vi "processCmd.vi"(8 "error in (no error)":errorcluster, 10 "tcpPacket":T1, 11 "tcpServerCmd in":refnum<class "TcpServerCmd.lvclass">) -> (0 "error out":errorcluster, 3 "tcpServerCmd out":refnum<class "TcpServerCmd.lvclass">)   [LabVIEW 2018, in "TcpServerCmd.lvclass"]
doc: "Process the incoming command."
uses:
  TcpServerCmd.lvclass
  home/pcortes/github/ts_labview_tcp_json/src/TcpServerBase/TcpServerBase.lvclass
  TcpServerBase/typedef/tcpPacketTypeDef.ctl
  TcpServerBase/TcpServerBase.lvclass/TcpServerBase.ctl
  TcpServerCmd.lvclass/TcpServerCmd.ctl
  TcpServerBase/TcpServerBase.lvclass
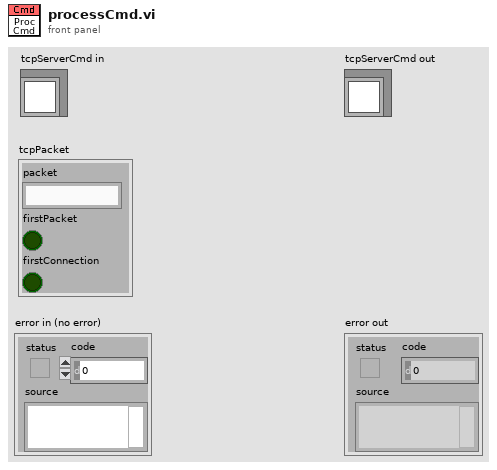
[diagram p1: front panel]
types:
  T1 = typedef "TcpServerBase.lvclass/tcpPacketTypeDef.ctl" = cluster{"packet":string, "firstPacket":bool, "firstConnection":bool}
  T2 = typedef "TcpServerCmd.lvclass/userEventTypeDef.ctl" = cluster{"CmdRead":refnum<user-event>, "CmdWrite":refnum<user-event>, "MsgRead":refnum<user-event>, "MsgWrite":refnum<user-event>, "GenRead":refnum<user-event>, "GenWrite":refnum<user-event>}
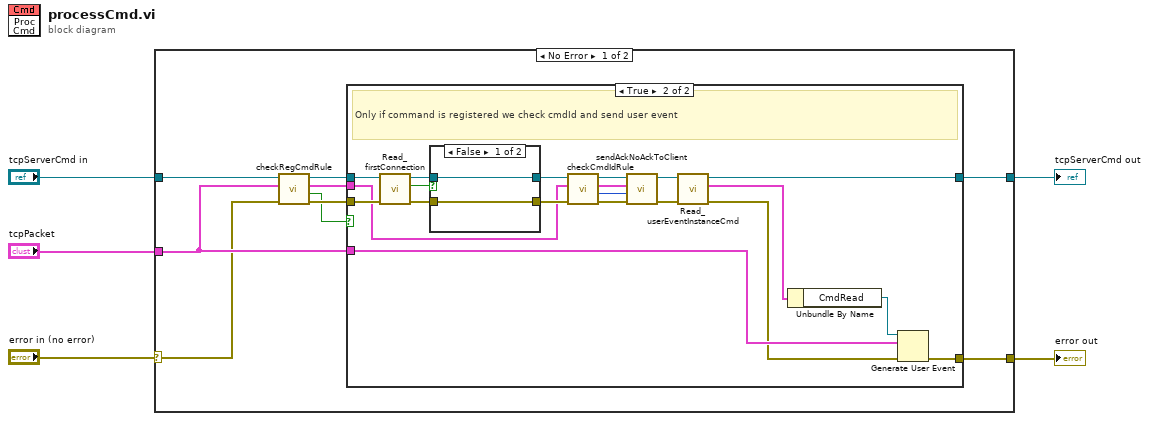
[diagram p0: block diagram]
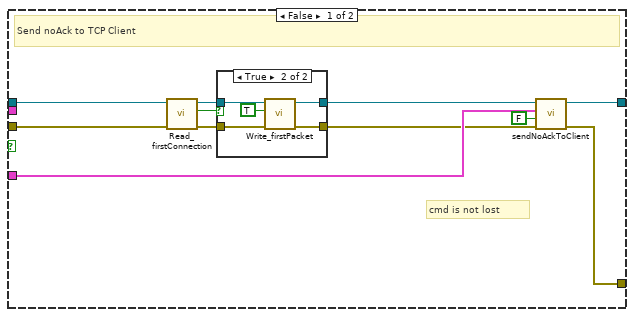
[diagram p2: hidden frame]
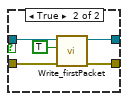
[diagram p4: hidden frame]
diagram:
  n1 = case shown="No Error" "error in (no error)" {
    selector: "error in (no error)" -> [w8 w61]
    tunnel: [w6 w61] -> w4
    tunnel: [w7 w60] -> w2
    tunnel: "tcpServerCmd in" -> [w10 w60]
    tunnel: "tcpPacket" -> [w9 _]
    frame No Error {
      n2 = call "checkRegCmdRule.vi"("error in (no error)"=w8, "tcpPacket"=w9, "tcpServerCmd in"=w10) -> ("error out"=w12:errorcluster, "regCmd?"=w11:bool, "tcpPacket"=w13:T1, "tcpServerCmd out"=w14:refnum<class "TcpServerCmd.lvclass">)  [unwired: 5 in]
      n3 = case shown="True" w11 {
        tunnel: [w24 w50] -> w7
        tunnel: [w25 w49] -> w6
        tunnel: w9 -> [w23 w48]
        tunnel: w14 -> [w22 w38]
        tunnel: w13 -> [_ w33]
        tunnel: w12 -> [w18 w40]
        frame False {
          # "cmd is not lost"
          # "Send noAck to TCP Client"
          n4 = call "Read_firstConnection.vi"("error in (no error)"=w18, "TcpServerBase in"=w22) -> ("error out"=w19:errorcluster, "firstConnection"=w20:bool, "TcpServerBase out"=w21:refnum<class "TcpServerCmd.lvclass">)  [unwired: 7 in]
          n5 = case shown="True" w20 {
            tunnel: w19 -> [w26 w32]
            tunnel: [w26 w31] -> w16
            tunnel: w21 -> [w27 w30]
            tunnel: [w27 w29] -> w17
            frame False {
            }
            frame True {
              n6 = call "Write_firstPacket.vi"("error in (no error)"=w32, "firstPacket"=TRUE, "TcpServerBase in"=w30) -> ("error out"=w31:errorcluster, "TcpServerBase out"=w29:refnum<class "TcpServerCmd.lvclass">)  [unwired: 7 in]
            }
          }
          n7 = call "sendNoAckToClient.vi"("error in (no error)"=w16, "cmdLost"=FALSE, "tcpPacket"=w23, "tcpServerCmd in"=w17) -> ("error out"=w25:errorcluster, "tcpServerCmd out"=w24:refnum<class "TcpServerCmd.lvclass">)  [unwired: 6 in]
        }
        frame True {
          # "Only if command is registered we check cmdId and send user event"
          n8 = call "Read_firstConnection.vi"("error in (no error)"=w40, "TcpServerBase in"=w38) -> ("error out"=w39:errorcluster, "firstConnection"=w34:bool, "TcpServerBase out"=w36:refnum<class "TcpServerCmd.lvclass">)  [unwired: 7 in]
          n9 = case shown="False" w34 {
            tunnel: w39 -> [w53 w59]
            tunnel: [w53 w58] -> w37
            tunnel: w36 -> [w54 w57]
            tunnel: [w54 w56] -> w35
            frame False {
            }
            frame True {
              n10 = call "Write_firstPacket.vi"("error in (no error)"=w59, "firstPacket"=TRUE, "TcpServerBase in"=w57) -> ("error out"=w58:errorcluster, "TcpServerBase out"=w56:refnum<class "TcpServerCmd.lvclass">)  [unwired: 7 in]
            }
          }
          n11 = call "checkCmdIdRule.vi"("error in (no error)"=w37, "tcpPacket"=w33, "tcpServerCmd in"=w35) -> ("error out"=w46:errorcluster, "ackIterations"=w45:i32, "tcpPacket"=w44:T1, "tcpServerCmd out"=w47:refnum<class "TcpServerCmd.lvclass">)  [unwired: 5 in]
          n12 = call "sendAckNoAckToClient.vi"("error in (no error)"=w46, "ackIterations"=w45, "tcpPacket"=w44, "tcpServerCmd in"=w47) -> ("error out"=w51:errorcluster, "tcpServerCmd out"=w52:refnum<class "TcpServerCmd.lvclass">)  [unwired: 6 in]
          n13 = call "Read_userEventInstanceCmd.vi"("error in (no error)"=w51, "TcpServerCmd in"=w52) -> ("error out"=w41:errorcluster, "userEventInstanceCmd"=w42:T2, "TcpServerCmd out"=w50:refnum<class "TcpServerCmd.lvclass">)  [unwired: 7 in]
          n14 = Unbundle By Name(w42) -> ("CmdRead"=w43:refnum<user-event>)
          n15 = Generate User Event(user event=w43, event data cluster=w48, error in=w41) -> (error out=w49:errorcluster)  [unwired: 1 in, 1 out]
        }
      }
    }
    frame Error {
    }
  }
  "error out" <- w4
  "tcpServerCmd out" <- w2
